vi "UHR-Fleezers Control (host) -Leonardo 04-2018 V1.vi"(0 "Tab Control":T5(tab)=enum."Trap Control (RF)") -> ()   [LabVIEW 2013] (continued)
                workers-P: _ -> [_]
                n1854 = Add Array Elements(numeric array=w3564) -> (sum=w3563:dbl)
              }
              n1855 = Select(t=w3550, s=w3551, f=w3549) -> (s? t:f=w3548:dbl)
              n1856 = Divide(x=w3555, y=w3548) -> (x/y=w3553:dbl[])
              n1857 = Bundle By Name(cluster=w3554, "magnitude"=w3553) -> (w3552:cluster{"f0":dbl, "df":dbl, "magnitude":dbl[]})
            }
          }
        }
        n1858 = case shown="True" w3494 {
          tunnel: w3495 -> [w3526 w3532]
          tunnel: [w3526 w3527] -> w3493
          frame False {
          }
          frame True {
            n1859 = Array Subset(array=w3532, index (row)=0 ("index"), length (row)=4 ("length"), index (col)=0 ("index"), length (col)=1 ("length")) -> (w3527:T47)
          }
        }
        n1860 = feedback-in #9(w3493) -> ()
        n1861 = Split 1D Array(array=w3507, index=2) -> (first subarray=→"FFT 1":cluster{"f0":dbl, "df":dbl, "magnitude":dbl[]}[], second subarray=→"FFT 2":cluster{"f0":dbl, "df":dbl, "magnitude":dbl[]}[])
      }
    }
    n1862 = Index Array(array=w2389, index=1) -> (element=w2397:waveform(dbl))
    n1863 = case "For displaying the high resolution display (no downsampling)" shown="True" w2453 {
      tunnel: w2416 -> [_ w2735]
      frame False {
      }
      frame True {
        n1864 = Index Array(array=w2735, index="High Res. Display") -> (element=w2736:waveform(dbl))
        n1865 = call <vilib>:"Std Deviation and Variance.vi"("X"=w2736) -> ("mean"=w2743:dbl, "standard deviation"=w2748:dbl)  [unwired: 1 in, 1 out]
        "Mean Intensity" <- w2743
        "Sigma" <- w2748
        n1866 = Subtract(x=w2736, y=w2743) -> (x-y=w2742:waveform(dbl))
        n1867 = Select(t=w2742, s="Subtract mean", f=w2736) -> (s? t:f=→"1 Channel":waveform(dbl))
        n1868 = Divide(x=w2748, y=w2743) -> (x/y=→"Sigma/Mean":dbl)
        n1869 = feedback #10(1) -> (w2737:i32)
        n1870 = Greater Or Equal?(x=w2737, y="Slow mean N ave.") -> (x >= y?=w2750:bool)
        n1871 = Increment(x=w2737) -> (x+1=w2752:i32)
        n1872 = Select(t=1, s=w2750, f=w2752) -> (s? t:f=w2739:i32)
        n1873 = feedback-in #10(w2739) -> ()
        n1874 = feedback #11() -> (w2740:waveform(dbl))  [unwired: 1 out]
        n1875 = case shown="Default" w2737 {
          tunnel: [w2755 w2758] -> w2741
          tunnel: w2740 -> [w2757 _]
          tunnel: w2736 -> [w2756 w2758]
          frame Default {
            n1876 = call-poly <vilib>:"Append Waveforms.vi"("waveform B"=w2756, "waveform A"=w2757) -> ("waveform out"=w2755:waveform(dbl))  [unwired: 1 in, 8 out]
          }
          frame 1 {
          }
        }
        n1877 = feedback-in #11(w2741) -> ()
        n1878 = case shown="True" w2750 {
          tunnel: w2741 -> [_ w2754]
          frame False {
          }
          frame True {
            n1879 = call-poly <vilib>:"Mean.vi"("X"=w2754) -> ("mean"=→"Slow mean":dbl)  [unwired: 1 out]
          }
        }
      }
    }
    n1880 = case "For plotting results of scanning MCL" shown="True" w2523 {
      tunnel: w2522 -> [_ w2875]
      tunnel: w2446 -> [_ w2971]
      tunnel: w2531 -> [_ _]
      tunnel: w2416 -> [_ w2945]
      tunnel: w2391 -> [_ w2876]
      tunnel: w2390 -> [_ w2849]
      frame False {
      }
      frame True {
        w2856 = u32 0 items=["Horizontal", "Vertical", "Central", "1st Diagonal", "2nd Diagonal"] ("Type of Symmetry")
        w2884 = u32 0 items=["Horizontal", "Vertical", "Central", "1st Diagonal", "2nd Diagonal"] ("Type of Symmetry")
        w2887 = u32 0 items=["Horizontal", "Vertical", "Central", "1st Diagonal", "2nd Diagonal"] ("Type of Symmetry")
        w2916 = u32 0 items=["Horizontal", "Vertical", "Central", "1st Diagonal", "2nd Diagonal"] ("Type of Symmetry")
        n1881 = Index Array(array=w2945, index=10) -> (element=w2951:waveform(dbl))
        n1882 = Index Array(array=w2945, index=11) -> (element=w2948:waveform(dbl))
        n1883 = local read "Cycles/step (MCL)"() -> (w2901:u64)
        n1884 = Index Array(array=w2945, index="Channel") -> (element=w2947:waveform(dbl))
        n1885 = Unbundle(w2849) -> ("New Image"=w2848:T3, "New Image"=w2847:T3, "New Image"=w2846:T3, "New Image"=w2845:T3)
        n1886 = Unbundle By Name(w2951) -> ("Y"=w2903:dbl[])
        n1887 = Unbundle By Name(w2948) -> ("Y"=w2905:dbl[])
        n1888 = Unbundle By Name(w2947) -> ("Y"=w2910:dbl[])
        n1889 = call "downsample 1D array - double.vi"("Ave N"=w2901, "Array In"=w2903) -> ("Array Out"=w2902:dbl[])  [unwired: 1 out]
        n1890 = call "downsample 1D array - double.vi"("Ave N"=w2901, "Array In"=w2905) -> ("Array Out"=w2904:dbl[])  [unwired: 1 out]
        n1891 = call "downsample 1D array - double.vi"("Ave N"=w2901, "Array In"=w2910) -> ("Array Out"=w2909:dbl[])  [unwired: 1 out]
        n1892 = feedback #12(w2971) -> (w2972:dbl[])
        n1893 = Build Array (concatenate)(w2972, w2971) -> (w2953:dbl[])
        n1894 = feedback #13(w2876) -> (w2878:dbl[])
        n1895 = Build Array (concatenate)(w2878, w2876) -> (w2877:dbl[])
        n1896 = local read "Scan steps (MCL)"() -> (w2858:u64)
        n1897 = Select(t=w2971, s=w2875, f=w2953) -> (s? t:f=w2957:dbl[])
        n1898 = feedback-in #12(w2957) -> ()
        n1899 = Select(t=w2876, s=w2875, f=w2877) -> (s? t:f=w2859:dbl[])
        n1900 = feedback-in #13(w2859) -> ()
        n1901 = local read "Scan lines (y)"() -> (w2844:u64)
        n1902 = local read "N APD Samp/step"() -> (w2860:dbl)
        n1903 = feedback #14(w2902) -> (w2959:dbl[])
        n1904 = Build Array (concatenate)(w2959, w2902) -> (w2950:dbl[])
        n1905 = feedback #15(w2909) -> (w2969:dbl[])
        n1906 = Build Array (concatenate)(w2969, w2909) -> (w2968:dbl[])
        n1907 = feedback #16(w2904) -> (w2961:dbl[])
        n1908 = Build Array (concatenate)(w2961, w2904) -> (w2962:dbl[])
        n1909 = Select(t=w2902, s=w2875, f=w2950) -> (s? t:f=w2906:dbl[])
        n1910 = feedback-in #14(w2906) -> ()
        n1911 = Select(t=w2909, s=w2875, f=w2968) -> (s? t:f=w2908:dbl[])
        n1912 = feedback-in #15(w2908) -> ()
        n1913 = Select(t=w2904, s=w2875, f=w2962) -> (s? t:f=w2907:dbl[])
        n1914 = feedback-in #16(w2907) -> ()
        n1915 = Multiply(x=w2858, y=u64 2) -> (x*y=w2843:u64)
        n1916 = call "integrate 1D array interval - double.vi"("Ave N"=w2860, "Array In"=w2859) -> ("Array Out"=w2871:dbl[])  [unwired: 1 out]
        n1917 = call "integrate 1D array interval - double.vi"("Ave N"=w2860, "Array In"=w2957) -> ("Array Out"=w2956:dbl[])  [unwired: 1 out]
        n1918 = Array Size(array=w2871) -> (size(s)=w2872:i32)
        n1919 = Array Size(array=w2956) -> (size(s)=w2958:i32)
        n1920 = Multiply(x=w2844, y=w2843) -> (x*y=w2874:u64)
        n1921 = Multiply(x=w2844, y=w2843) -> (x*y=w2966:u64)
        n1922 = call-poly <vilib>:"Mean.vi"("X"=w2906) -> ("mean"=w2890:dbl)  [unwired: 1 out]
        n1923 = Subtract(x=w2874, y=w2872) -> (x-y=w2865:u64)
        n1924 = call-poly <vilib>:"Mean.vi"("X"=w2908) -> ("mean"=w2895:dbl)  [unwired: 1 out]
        n1925 = call-poly <vilib>:"Mean.vi"("X"=w2907) -> ("mean"=w2893:dbl)  [unwired: 1 out]
        n1926 = call-poly <vilib>:"Mean.vi"("X"=w2871) -> ("mean"=w2862:dbl)  [unwired: 1 out]
        n1927 = Subtract(x=w2966, y=w2958) -> (x-y=w2900:u64)
        n1928 = call-poly <vilib>:"Mean.vi"("X"=w2956) -> ("mean"=w2897:dbl)  [unwired: 1 out]
        n1929 = Initialize Array(1.0 ("element"), w2865) -> (w2861:dbl[])
        n1930 = Initialize Array(1.0 ("element"), w2900) -> (w2891:dbl[])
        n1931 = Multiply(x=w2861, y=w2862) -> (x*y=w2863:dbl[])
        n1932 = Multiply(x=w2891, y=w2893) -> (x*y=w2894:dbl[])
        n1933 = Multiply(x=w2891, y=w2895) -> (x*y=w2896:dbl[])
        n1934 = Multiply(x=w2891, y=w2890) -> (x*y=w2892:dbl[])
        n1935 = Multiply(x=w2891, y=w2897) -> (x*y=w2898:dbl[])
        n1936 = Build Array (concatenate)(w2906, w2892) -> (w2960:dbl[])
        n1937 = Build Array (concatenate)(w2908, w2896) -> (w2964:dbl[])
        n1938 = Build Array (concatenate)(w2907, w2894) -> (w2963:dbl[])
        n1939 = Build Array (concatenate)(w2871, w2863) -> (w2873:dbl[])
        n1940 = Build Array (concatenate)(w2956, w2898) -> (w2965:dbl[])
        n1941 = Reshape Array(w2960, w2844, w2843) -> (w2926:dbl[][])
        n1942 = Reshape Array(w2873, w2844, w2843) -> (w2869:dbl[][])
        n1943 = Reshape Array(w2964, w2844, w2843) -> (w2918:dbl[][])
        n1944 = Reshape Array(w2963, w2844, w2843) -> (w2933:dbl[][])
        n1945 = Reshape Array(w2965, w2844, w2843) -> (w2943:dbl[][])
        n1946 = Array Subset(array=w2933, index (col)=0 ("index"), length (col)=w2858) -> (w2938:dbl[][])  [unwired: 2 in]
        n1947 = Array Subset(array=w2933, index (col)=w2858) -> (w2936:dbl[][])  [unwired: 3 in]
        n1948 = Array Subset(array=w2918, index (col)=0 ("index"), length (col)=w2858) -> (w2924:dbl[][])  [unwired: 2 in]
        n1949 = Array Subset(array=w2918, index (col)=w2858) -> (w2922:dbl[][])  [unwired: 3 in]
        n1950 = Array Subset(array=w2869, index (col)=0 ("index"), length (col)=w2858) -> (w2868:dbl[][])  [unwired: 2 in]
        n1951 = Array Subset(array=w2869, index (col)=w2858) -> (w2866:dbl[][])  [unwired: 3 in]
        n1952 = Array Subset(array=w2943, index (col)=0 ("index"), length (col)=w2858) -> (w2942:dbl[][])  [unwired: 2 in]
        n1953 = Array Subset(array=w2943, index (col)=w2858) -> (w2940:dbl[][])  [unwired: 3 in]
        n1954 = Array Subset(array=w2926, index (col)=0 ("index"), length (col)=w2858) -> (w2931:dbl[][])  [unwired: 2 in]
        n1955 = Array Subset(array=w2926, index (col)=w2858) -> (w2929:dbl[][])  [unwired: 3 in]
        n1956 = for {
          tunnel: w2938 -> [w2980] mode=indexing
          tunnel: [w2979] -> w2937 mode=indexing
          workers-P: _ -> [_]
          n1957 = Reverse 1D Array(array=w2980) -> (reversed array=w2979:dbl[])
        }
        n1958 = for {
          tunnel: w2924 -> [w2976] mode=indexing
          tunnel: [w2975] -> w2923 mode=indexing
          workers-P: _ -> [_]
          n1959 = Reverse 1D Array(array=w2976) -> (reversed array=w2975:dbl[])
        }
        n1960 = for {
          tunnel: w2868 -> [w2974] mode=indexing
          tunnel: [w2973] -> w2867 mode=indexing
          workers-P: _ -> [_]
          n1961 = Reverse 1D Array(array=w2974) -> (reversed array=w2973:dbl[])
        }
        n1962 = for {
          tunnel: w2942 -> [w2982] mode=indexing
          tunnel: [w2981] -> w2941 mode=indexing
          workers-P: _ -> [_]
          n1963 = Reverse 1D Array(array=w2982) -> (reversed array=w2981:dbl[])
        }
        n1964 = for {
          tunnel: w2931 -> [w2978] mode=indexing
          tunnel: [w2977] -> w2930 mode=indexing
          workers-P: _ -> [_]
          n1965 = Reverse 1D Array(array=w2978) -> (reversed array=w2977:dbl[])
        }
        n1966 = Index Array(array=w2943, index (row)=0) -> (element=→"Waveform Graph":dbl[])  [unwired: 1 in]
        n1967 = Add(x=w2937, y=w2936) -> (x+y=w2935:dbl[][])
        n1968 = Add(x=w2923, y=w2922) -> (x+y=w2921:dbl[][])
        n1969 = Add(x=w2867, y=w2866) -> (x+y=w2851:dbl[][])
        n1970 = Add(x=w2941, y=w2940) -> (x+y=w2915:dbl[][])
        n1971 = Add(x=w2930, y=w2929) -> (x+y=w2928:dbl[][])
        n1972 = Divide(x=w2921, y=2) -> (x/y=w2919:dbl[][])
        n1973 = Divide(x=w2935, y=2) -> (x/y=w2880:dbl[][])
        n1974 = Divide(x=w2928, y=2) -> (x/y=w2882:dbl[][])
        n1975 = To Single Precision Float(number=w2915) -> (single precision float=w2914:sgl[][])
        n1976 = Transpose 2D Array(2D array=w2919) -> (transposed array=→"Data map":dbl[][])
        n1977 = To Single Precision Float(number=w2851) -> (single precision float=w2855:sgl[][])
        n1978 = To Single Precision Float(number=w2880) -> (single precision float=w2886:sgl[][])
        n1979 = To Single Precision Float(number=w2882) -> (single precision float=w2883:sgl[][])
        n1980 = call "IMAQ ArrayToImage"("Image Pixels (Float)"=w2914, "Image"=w2848) -> ("Image Out"=w2917:T3)  [unwired: 8 in, 1 out]
        n1981 = call "IMAQ ArrayToImage"("Image Pixels (Float)"=w2855, "Image"=w2847) -> ("Image Out"=w2857:T3)  [unwired: 8 in, 1 out]
        n1982 = call "IMAQ ArrayToImage"("Image Pixels (Float)"=w2886, "Image"=w2846) -> ("Image Out"=w2888:T3)  [unwired: 8 in, 1 out]
        n1983 = call "IMAQ ArrayToImage"("Image Pixels (Float)"=w2883, "Image"=w2845) -> ("Image Out"=w2885:T3)  [unwired: 8 in, 1 out]
        n1984 = call "IMAQ Symmetry"("Type of Symmetry"=w2916, "Image Src"=w2917) -> ("Image Dst Out"=w2912:T3)  [unwired: 3 in, 1 out]
        n1985 = call "IMAQ Symmetry"("Type of Symmetry"=w2856, "Image Src"=w2857) -> ("Image Dst Out"=w2853:T3)  [unwired: 3 in, 1 out]
        n1986 = call "IMAQ Symmetry"("Type of Symmetry"=w2887, "Image Src"=w2888) -> ("Image Dst Out"=→"Detection Laser X":T3)  [unwired: 3 in, 1 out]
        n1987 = call "IMAQ Symmetry"("Type of Symmetry"=w2884, "Image Src"=w2885) -> ("Image Dst Out"=→"Detection Laser Y":T3)  [unwired: 3 in, 1 out]
        n1988 = call "IMAQ Set Simple Calibration"("Calibration Axis Info"=T37 {"Origin Pixel"={"X"=0.0, "Y"=0.0}, "Angle Relative to Horizontal (deg)"=0.0, "Axis Reference"=0}, "Grid Descriptor"=T38 {"X Step"=0.3, "Y Step"=0.3, "Unit"=enum."Undefined"}, "Image"=w2912) -> ("Calibrated Image"=→"APD 1":T3)  [unwired: 7 in, 1 out]
        n1989 = call "IMAQ Set Simple Calibration"("Calibration Axis Info"=T37 {"Origin Pixel"={"X"=0.0, "Y"=0.0}, "Angle Relative to Horizontal (deg)"=0.0, "Axis Reference"=0}, "Grid Descriptor"=T38 {"X Step"=0.3, "Y Step"=0.3, "Unit"=enum."Undefined"}, "Image"=w2853) -> ("Calibrated Image"=→"APD 2":T3)  [unwired: 7 in, 1 out]
      }
    }
    n1990 = Subtract(x=w2397, y="APD 2 Offset") -> (x-y=w2394:waveform(dbl))
    n1991 = Subtract(x=w2399, y="APD 1 Offset") -> (x-y=w2395:waveform(dbl))
    n1992 = Index Array(array=w2414, index=3) -> (element=w2473:waveform(dbl))
    n1993 = Index Array(array=w2414, index=6) -> (element=w2470:waveform(dbl))
    n1994 = Build Array(w2395, w2394) -> (→"APD Chart":waveform(dbl)[])
    n1995 = Array Size(array=w2463) -> (size(s)=w2511:i32)
    n1996 = call <vilib>:"Std Deviation and Variance.vi"("X"=w2407) -> ("standard deviation"=w2406:dbl)  [unwired: 1 in, 2 out]
    n1997 = Add Array Elements(numeric array=w2407) -> (sum=w2409:u32)
    n1998 = Add Array Elements(numeric array=w2463) -> (sum=w2521:u32)
    n1999 = call <vilib>:"Std Deviation and Variance.vi"("X"=w2463) -> ("standard deviation"=w2462:dbl)  [unwired: 1 in, 2 out]
    n2000 = Divide(x=w2406, y=w2405) -> (x/y=w2402:dbl)
    "Rate sigma (Hz) 2" <- w2402
    n2001 = Multiply(x=w2405, y=w2511) -> (x*y=w2408:dbl)
    "Int. Time (s)" <- w2408
    n2002 = Divide(x=w2409, y=w2408) -> (x/y=w2403:dbl)
    "APD 2 Rate (Hz)" <- w2403
    n2003 = Divide(x=w2521, y=w2408) -> (x/y=w2460:dbl)
    "APD 1 Rate (Hz)" <- w2460
    n2004 = Divide(x=w2462, y=w2405) -> (x/y=w2461:dbl)
    "Rate sigma (Hz)" <- w2461
    n2005 = Divide(x=w2402, y=w2403) -> (x/y=→"Sigma/Mean 2":dbl)
    n2006 = Divide(x=w2461, y=w2460) -> (x/y=→"Sigma/Mean":dbl)
    n2007 = case shown="2" "Calibration" {
      tunnel: "T1 alpha_x (nm/V)" -> [_ w2811 w2832]
      tunnel: "T1 kappa_x (pN/nm)" -> [_ _ w2822]
      tunnel: "T2 alpha_x (nm/V)" -> [_ w2810 w2830]
      tunnel: "T2 kappa_x (pN/nm)" -> [_ _ w2823]
      tunnel: w2473 -> [w2793 w2808 w2828]
      tunnel: w2470 -> [w2792 w2806 w2826]
      tunnel: [w2793 w2805 w2825] -> w2263
      tunnel: [w2792 w2804 w2824] -> w2269
      tunnel: ["T1 X (V)" ("Label.Text") "T1 X (nm)" ("Label.Text") "T1 X (pN)" ("Label.Text")] -> w2491
      tunnel: ["T2 X (V)" ("Label.Text") "T2 X (nm)" ("Label.Text") "T2 X (pN)" ("Label.Text")] -> w2490
      tunnel: ["Position (V)" ("Label.Text") "Position (nm)" ("Label.Text") "Force (pN)" ("Label.Text")] -> w2492
      tunnel: w2472 -> [_ w2796 w2815]
      tunnel: w2474 -> [_ w2799 w2817]
      tunnel: ["Mean (V)" ("Label.Text") "Mean (nm)" ("Label.Text") "Mean (pN)" ("Label.Text")] -> w2487
      tunnel: ["Difference (V)" ("Label.Text") "Difference (nm)" ("Label.Text") "Difference (pN)" ("Label.Text")] -> w2422
      frame 0, Default {
      }
      frame 1 {
        # "position"
        n2008 = Unbundle By Name(w2808) -> ("Y"=w2812:dbl[])
        n2009 = Unbundle By Name(w2806) -> ("Y"=w2797:dbl[])
        n2010 = Subtract(x=w2812, y=w2799) -> (x-y=w2800:dbl[])
        n2011 = Subtract(x=w2797, y=w2796) -> (x-y=w2798:dbl[])
        n2012 = Multiply(x=w2798, y=w2810) -> (x*y=w2807:dbl[])
        n2013 = Multiply(x=w2811, y=w2800) -> (x*y=w2809:dbl[])
        n2014 = Bundle By Name(cluster=w2806, "Y"=w2807) -> (w2804:waveform(dbl))
        n2015 = Bundle By Name(cluster=w2808, "Y"=w2809) -> (w2805:waveform(dbl))
      }
      frame 2 {
        # "force"
        n2016 = Unbundle By Name(w2828) -> ("Y"=w2833:dbl[])
        n2017 = Unbundle By Name(w2826) -> ("Y"=w2831:dbl[])
        n2018 = Subtract(x=w2831, y=w2815) -> (x-y=w2816:dbl[])
        n2019 = Subtract(x=w2833, y=w2817) -> (x-y=w2818:dbl[])
        n2020 = Compound Arithmetic op=MULTIPLY(w2816, w2830, w2823) -> (w2827:dbl[])
        n2021 = Compound Arithmetic op=MULTIPLY(w2822, w2832, w2818) -> (w2829:dbl[])
        n2022 = Bundle By Name(cluster=w2826, "Y"=w2827) -> (w2824:waveform(dbl))
        n2023 = Bundle By Name(cluster=w2828, "Y"=w2829) -> (w2825:waveform(dbl))
      }
    }
    n2024 = feedback-in #17("Calibration") -> ()
    n2025 = feedback #17(u16 1 ("Calibration")) -> (w2494:u16)
    n2026 = local read "Trap 2 Bead Size (nm)"() -> (w2302:dbl)
    n2027 = local read "Trap 1 Bead Size (nm)"() -> (w2301:dbl)
    n2028 = local read "AOM X Cal (nm/MHz)"() -> (w2299:dbl)
    n2029 = local read "Trap Delta (MHz)"() -> (w2298:dbl)
    n2030 = Not Equal?(x=w2494, y="Calibration") -> (x != y?=w2451:bool)
    n2031 = Multiply(x=w2299, y=w2298) -> (x*y=w2303:dbl)
    n2032 = Unbundle By Name(w2263) -> ("Y"=w2268:dbl[])
    n2033 = Unbundle By Name(w2269) -> ("Y"=w2267:dbl[])
    n2034 = Add(x=w2302, y=w2301) -> (x+y=w2305:dbl)
    n2035 = case shown="False" "Negate trap 2 force" {
      tunnel: [-1.0 1.0] -> w2480
      frame False {
      }
      frame True {
      }
    }
    n2036 = Unbundle By Name(w2473) -> ("Y"=w2476:dbl[])
    n2037 = Unbundle By Name(w2470) -> ("Y"=w2479:dbl[])
    n2038 = Divide(x=w2305, y=2.0) -> (x/y=w2300:dbl)
    n2039 = Subtract(x=w2268, y=w2267) -> (x-y=w2265:dbl[])
    n2040 = Subtract(x=w2476, y=w2474) -> (x-y=w2477:dbl[])
    n2041 = Subtract(x=w2479, y=w2472) -> (x-y=w2478:dbl[])
    n2042 = Divide(x=w2265, y=2.0) -> (x/y=w2264:dbl[])
    n2043 = Multiply(x=w2478, y="T2 alpha_x (nm/V)") -> (x*y=w2469:dbl[])
    n2044 = Multiply(x="T1 alpha_x (nm/V)", y=w2477) -> (x*y=w2468:dbl[])
    n2045 = Multiply(x=w2269, y=w2480) -> (x*y=w2481:waveform(dbl))
    n2046 = Bundle By Name(cluster=w2263, "Y"=w2264) -> (w2262:waveform(dbl))
    n2047 = case shown="True" "Read Lateness and Rel Phase" {
      tunnel: w2275 -> [w2759 w2781]
      tunnel: w2314 -> [w2760 w2780]
      tunnel: [w2759 w2779] -> w2466
      tunnel: [w2760 w2778] -> w2465
      frame False {
      }
      frame True {
        n2048 = xnode "Read/Write Control"("FPGA VI Reference In"=w2781, "error in"=w2780) -> ("FPGA VI Reference Out"=w2779:T20, "error out"=w2778:errorcluster, "GI Relative phase"=→"GI relative phase":i16, "Relative phase"=→"Relative phase (AI1)":i16, "AI Late Counter"=→"Late Counter (AI1)":u8, "GI Late Counter"=→"GI Late Counter":u8, "MCL Late Counter"=→"MCL Late Counter":u8, "MCL Relative Phase"=→"Relative Phase (MCL)":i16, "APD Acq Relative Phase"=→"APD Acq Relative Phase":i16, "APD 1 Gate Relative Phase"=→"APD 1 Gate Relative Phase":i16, "APD 2 Gate Relative Phase"=→"APD 2 Gate Relative Phase":i16, "APD Acq Late Counter"=→"APD Acq Late Counter":u16, "APD 1 Gate Late Counter"=→"APD 1 Gate Late Counter":u8, "APD 2 Gate Late Counter"=→"APD 2 Gate Late Counter":u8, "Green FB Relative Phase"=→"Relative phase (Green FB)":i16, "GI Relative phase"=→"GI relative phase 2":i16, "GI Late Counter 2"=→"GI Late Counter 2":u16, "Trap Pos FIFO Timeout"=→"Trap Pos FIFO Timeout":u16, "Trap AI FIFO Timeout"=→"Trap AI FIFO Timeout":u16)
      }
    }
    n2049 = Subtract(x=w2469, y=w2468) -> (x-y=w2297:dbl[])
    n2050 = call-poly <vilib>:"Mean.vi"("X"=w2297) -> ("mean"=w2304:dbl)  [unwired: 1 out]
    n2051 = Add(x=w2303, y=w2304) -> (x+y=w2307:dbl)
    n2052 = Subtract(x=w2307, y=w2300) -> (x-y=→"Tether Extension (nm, calculated)":dbl)
    n2053 = Unbundle By Name(w2269) -> ("Y"=w2260:dbl[])
    n2054 = Unbundle By Name(w2263) -> ("Y"=w2261:dbl[])
    n2055 = Build Array(w2263, w2481, w2262) -> (→"Force":waveform(dbl)[])
    n2056 = Subtract(x=w2297, y="Offset (nm)") -> (x-y=w2441:dbl[])
    n2057 = call-poly <vilib>:"Mean.vi"("X"=w2260) -> ("mean"=w2258:dbl)  [unwired: 1 out]
    "T2 X" <- w2258
    n2058 = call-poly <vilib>:"Mean.vi"("X"=w2261) -> ("mean"=w2259:dbl)  [unwired: 1 out]
    "T1 X" <- w2259
    n2059 = Subtract(x=w2261, y=w2260) -> (x-y=w2443:dbl[])
    n2060 = Bundle By Name(cluster=w2473, "Y"=w2441) -> (w2413:waveform(dbl))
    "Bead Separation" <- w2413
    n2061 = Divide(x=w2443, y=2.0) -> (x/y=→"Vec Mean of T1 T2":dbl[])
    n2062 = case shown="True" w2451 {
      tunnel: w2492 -> [_ w2786]
      tunnel: w2491 -> [_ w2785]
      tunnel: w2490 -> [_ w2784]
      tunnel: w2487 -> [_ w2783]
      tunnel: w2422 -> [_ w2782]
      frame False {
      }
      frame True {
        n2063 = property on="Force" class="WFChart (strict)"("YScale.NameLbl.Text"=w2786) -> ()  [unwired: 2 in, 2 out]
        n2064 = property on="T2 X" class="DigNum (strict)"("Caption.Text"=w2784) -> ()  [unwired: 2 in, 2 out]
        n2065 = property on="T1 X" class="DigNum (strict)"("Caption.Text"=w2785) -> ()  [unwired: 2 in, 2 out]
        n2066 = property on="Mean" class="DigNum (strict)"("Caption.Text"=w2783) -> ()  [unwired: 2 in, 2 out]
        n2067 = property on="Difference" class="DigNum (strict)"("Caption.Text"=w2782) -> ()  [unwired: 2 in, 2 out]
      }
    }
    n2068 = local read "Tether"() -> (w2445:bool)
    n2069 = Subtract(x=w2259, y=w2258) -> (x-y=w2489:dbl)
    n2070 = Add(x=w2259, y=w2258) -> (x+y=→"Difference":dbl)
    n2071 = feedback #18(w2441) -> (w2440:dbl[])
    n2072 = Divide(x=w2489, y=2.0) -> (x/y=w2272:dbl)
    "Mean" <- w2272
    n2073 = case shown="True" w2445 {
      tunnel: w2272 -> [_ w2718]
      frame False {
      }
      frame True {
        n2074 = Greater?(x="Lost Tether Alarm Threshold (pN)", y=w2718) -> (0:w2716:bool)
        n2075 = case shown="True" w2716 {
          frame False {
          }
          frame True {
            n2076 = flat-sequence {
              frame #0 {
                # "stop only if saving"
                n2077 = local read "Saving..."() -> (w2731:bool)
                n2078 = And(x=w2731, y="TA Cancel Save?") -> (x .and. y?=w2730:bool)
                n2079 = local write "Stop Saving"(w2730) -> ()
              }
              frame #1 {
                n2080 = case shown="True" "TA Green Off?" {
                  frame False {
                  }
                  frame True {
                    w2734 = FALSE ("Fl. Triggered...")
                    n2081 = local write "Fl. Triggered..."(w2734) -> ()
                    n2082 = property on="Green Laser ON/Interlacing" class="Bool (strict)"("Val(Sgnl)"=w2734) -> ()  [unwired: 2 in, 2 out]
                  }
                }
              }
            }
            n2083 = local read "Time tether formed"() -> (w2725:timestamp)
            n2084 = Get Date/Time In Seconds() -> (seconds since 1Jan1904=w2726:timestamp)
            n2085 = Subtract(x=w2726, y=w2725) -> (x-y=w2724:dbl)
            n2086 = Number To Decimal String(number=w2724) -> (decimal integer string=w2721:string)  [unwired: 1 out]
            n2087 = local read "Messages"() -> (w2728:string)
            n2088 = call <vilib>:"Beep.vi"() -> ()  [unwired: 3 in, 9 out]
            n2089 = Concatenate Strings("Lost tether (" ("Message to add"), w2721, " s)." ("string")) -> (w2723:string)
            n2090 = local write "Tether"(FALSE ("Tether")) -> ()
            n2091 = call "Update messages.vi"("Message to add"=w2723, "Old message string"=w2728) -> ("New message string"=w2727:string)
            n2092 = local write "Messages"(w2727) -> ()
            n2093 = property on="Trap Pos. FB ON" class="Bool (strict)"("Val(Sgnl)"=FALSE ("Value (Signaling)")) -> ()  [unwired: 2 in, 2 out]
          }
        }
      }
    }
    n2094 = Build Array (concatenate)(w2441, w2440) -> (w2439:dbl[])
    n2095 = Split 1D Array(array=w2439, index=w2325) -> (first subarray=w2435:dbl[])  [unwired: 1 out]
    n2096 = feedback-in #18(w2435) -> ()
    n2097 = call-poly <vilib>:"Mean.vi"("X"=w2435) -> ("mean"=w2434:dbl)  [unwired: 1 out]
    "Bead Mean (nm)" <- w2434
    n2098 = Subtract(x=w2435, y=w2434) -> (x-y=w2433:dbl[])
    n2099 = Square(x=w2433) -> (x^2=w2432:dbl[])
    n2100 = case shown="True" "Semi Passive ON" {
      tunnel: "Semi Passive mode" -> [_ w2599]
      tunnel: "Jump Force (pN)" -> [_ w2598]
      tunnel: w2272 -> [_ w2597]
      frame False {
      }
      frame True {
        n2101 = case shown="\"Use Feedback\"" w2599 {
          tunnel: w2598 -> [_ w2602 w2618]
          tunnel: w2597 -> [_ w2601 w2617]
          frame "None" {
          }
          frame "Use Feedback" {
            n2102 = local read "Target Force (pN)"() -> (w2604:dbl)
            n2103 = Less?(x=w2602, y=w2604) -> (x < y?=w2603:bool)
            n2104 = case shown="True" w2603 {
              tunnel: w2602 -> [w2611 w2614]
              tunnel: w2601 -> [w2610 w2613]
              tunnel: [w2609 w2612] -> w2600
              frame False {
                n2105 = Less?(x=w2611, y=w2610) -> (x < y?=w2609:bool)
              }
              frame True {
                n2106 = Greater?(x=w2614, y=w2613) -> (0:w2612:bool)
              }
            }
            n2107 = case shown="True" w2600 {
              frame False {
                n2108 = local read "Trap Pos. FB ON"() -> (w2605:bool)
                n2109 = case shown="True" w2605 {
                  frame False {
                  }
                  frame True {
                    n2110 = property on="Trap Pos. FB ON" class="Bool (strict)"("Val(Sgnl)"=FALSE) -> ()  [unwired: 2 in, 2 out]
                  }
                }
              }
              frame True {
                n2111 = local read "Trap Pos. FB ON"() -> (w2607:bool)
                n2112 = case shown="False" w2607 {
                  frame False {
                    n2113 = property on="Trap Pos. FB ON" class="Bool (strict)"("Val(Sgnl)"=TRUE) -> ()  [unwired: 2 in, 2 out]
                  }
                  frame True {
                  }
                }
              }
            }
          }
          frame "Sharp Jump" {
            n2114 = local read "Target Force (pN)"() -> (w2620:dbl)
            n2115 = Greater?(x=w2618, y=w2620) -> (0:w2619:bool)
            n2116 = case shown="True" w2619 {
              tunnel: w2618 -> [w2635 w2639]
              tunnel: w2617 -> [w2636 w2638]
              tunnel: [w2634 w2637] -> w2616
              frame False {
                n2117 = Greater?(x=w2636, y=w2635) -> (0:w2634:bool)
              }
              frame True {
                n2118 = Less?(x=w2639, y=w2638) -> (x < y?=w2637:bool)
              }
            }
            n2119 = Subtract(x=w2618, y=w2620) -> (x-y=w2615:dbl)
            n2120 = case shown="True" w2616 {
              tunnel: w2615 -> [_ w2626]
              frame False {
              }
              frame True {
                n2121 = local read "T1 kappa_x (pN/nm)"() -> (w2631:dbl)
                n2122 = local read "T2 kappa_x (pN/nm)"() -> (w2632:dbl)
                n2123 = Reciprocal(x="DNA stiffness (pN / nm)") -> (1/x=w2628:dbl)
                n2124 = Reciprocal(x=w2631) -> (1/x=w2630:dbl)
                n2125 = Reciprocal(x=w2632) -> (1/x=w2629:dbl)
                n2126 = Compound Arithmetic op=ADD(w2630, w2629, w2628) -> (w2627:dbl)
                n2127 = local read "AOM X Cal (nm/MHz)"() -> (w2625:dbl)
                n2128 = Multiply(x=w2627, y=w2626) -> (x*y=w2624:dbl)
                n2129 = local read "Trap Delta (MHz)"() -> (w2622:dbl)
                n2130 = Divide(x=w2624, y=w2625) -> (x/y=w2623:dbl)
                n2131 = Subtract(x=w2622, y=w2623) -> (x-y=w2621:dbl)
                n2132 = property on="Trap Delta (MHz)" class="DigNum (strict)"("Val(Sgnl)"=w2621) -> ()  [unwired: 2 in, 2 out]
              }
            }
          }
        }
      }
    }
    n2133 = call-poly <vilib>:"Mean.vi"("X"=w2432) -> ("mean"=w2431:dbl)  [unwired: 1 out]
    n2134 = Square Root(x=w2431) -> (sqrt(x)=w2430:dbl)
    n2135 = Multiply(x=10.0, y=w2430) -> (x*y=→"RMS (Ang)":dbl)
    n2136 = xnode "Read/Write Control"("FPGA VI Reference In"=w2466, "error in"=w2465) -> ("FPGA VI Reference Out"=w2575:T20, "error out"=w2569:errorcluster, "AI2 Y Sum Set 1"=w2565:i16, "AI2 Y Sum Set 2"=w2564:i16, "AI1 X Set 1"=w2359:fxp<+/-,16,1>, "AI1 X Set 2"=w2358:fxp<+/-,16,1>, "Trap Pos FB Int Signal"=→"Trap Pos FB Int Signal":fxp<+/-,24,9>, "Trap Pos FB Int-Norm Signal"=→"Trap Pos FB Int-Norm Signal":fxp<+/-,16,1>, "Trap Pos FB Action"=w2352:i64, "Scanning"=→"AOD Scanning":bool, "Scan I"=→"AOD Scan I":u64, "Scanning MCL"=w2567:bool, "Scan I (MCL)"=→"MCL Scan I":u64, "Green FB Signals"=w2506:T48, "BD1 amplitude 1 out"=w2257:u16, "BD1 amplitude 2 out"=w2242:u16)  [unwired: 1 out]
    "MCL Scanning" <- w2567
    "Trap Pos FB Action" <- w2352
    n2137 = local read "AI2 (V)"() -> (w2566:cluster{"Set 1":dbl, "Set 2":dbl})
    n2138 = Bundle By Name(cluster=w2566, "Set 1"=w2565, "Set 2"=w2564) -> (w2562:cluster{"Set 1":dbl, "Set 2":dbl})
    n2139 = Divide(x=w2352, y=327.67) -> (x/y=→"Action (%)":dbl)
    n2140 = local read "Trap X (AI1)"() -> (w2372:T1)
    n2141 = Divide(x=w2562, y=3276.7) -> (x/y=w2561:cluster{"Set 1":dbl, "Set 2":dbl})
    n2142 = local write "AI2 (V)"(w2561) -> ()
    n2143 = Bundle(cluster=w2372, "Trap 1"=w2359, "Trap 2"=w2358) -> (→"Trap X (AI1)":T1)
    n2144 = Scale By Power Of 2(n=i16 12, x=ext 1.0) -> (x*2^n=w2253:ext)
    n2145 = Subtract(x=w2253, y=ext 1.0) -> (x-y=w2250:ext)
    n2146 = Divide(x=w2506, y=3276.7) -> (x/y=w2502:T49)
    n2147 = Multiply(x=w2257, y=ext 100.0) -> (x*y=w2251:ext)
    n2148 = Unbundle By Name(w2502) -> ("Green FB Ch 0"=w2505:dbl, "Green FB Ch 1"=w2504:dbl, "Green FB Ch 2"=w2503:dbl)
    n2149 = local read "All FB On/Off"() -> (w2241:bool)
    n2150 = Divide(x=w2251, y=w2250) -> (x/y=w2240:ext)
    "Trap 1 amplitude" <- w2240
    n2151 = Scale By Power Of 2(n=i16 12, x=ext 1.0) -> (x*2^n=w2246:ext)
    n2152 = Subtract(x=w2246, y=ext 1.0) -> (x-y=w2249:ext)
    n2153 = Multiply(x=w2242, y=ext 100.0) -> (x*y=w2248:ext)
    n2154 = Divide(x=w2505, y=w2503) -> (x/y=w2501:dbl)
    n2155 = Divide(x=w2504, y=w2503) -> (x/y=w2500:dbl)
    n2156 = flat-sequence "To save data" {
      tunnel: [w3615] -> w2586
      tunnel: [w3616] -> w2585
      tunnel: w2537 -> [w3609]
      tunnel: w2437 -> [w3613]
      tunnel: ["Save Calibration"] -> w2558
      tunnel: w2555 -> [w3612]
      tunnel: [w3605] -> w2554
      tunnel: [w3602] -> w2553
      tunnel: [w3599] -> w2552
      tunnel: w2536 -> [w3601]
      tunnel: w2449 -> [w3595]
      tunnel: [w3595] -> w2448
      tunnel: ["Start Saving"] -> w2415
      tunnel: [w3589] -> w2341
      tunnel: [w3588] -> w2340
      tunnel: w2586 -> [w3850]
      tunnel: w2585 -> [w3849]
      tunnel: w2342 -> [w3848]
      tunnel: w2558 -> [w3847]
      tunnel: w2554 -> [w3845]
      tunnel: w2553 -> [w3844]
      tunnel: w2552 -> [w3843]
      tunnel: w2424 -> [w3842]
      tunnel: w2458 -> [w3841]
      tunnel: w2448 -> [w3840]
      tunnel: w2415 -> [w3839]
      tunnel: w2413 -> [w3838]
      tunnel: w2389 -> [w3837]
      tunnel: w2341 -> [w3836]
      tunnel: w2340 -> [w3835]
      tunnel: w2339 -> [w3834]
      frame #0 {
        n2157 = Or(x="Save N Sets", y="Start Saving") -> (x .or. y?=w3596:bool)
        n2158 = To Double Precision Float(number=w3612) -> (double precision float=w3606:dbl)
        n2159 = Build Array(w3596, "Save Calibration", w3609, w3601) -> (w3611:bool[])
        n2160 = Compound Arithmetic op=OR("Save Calibration", w3609, w3596, w3601) -> (w3614:bool)
        n2161 = Boolean Array To Number(Boolean array=w3611) -> (number=w3608:u32)
        n2162 = feedback #19(FALSE ("Save APD Data\nwith Trap Data")) -> (w3590:bool)
        n2163 = feedback #20(refnum<k0> refnum) -> (w3617:refnum<file>)
        n2164 = feedback #21(refnum<k0> refnum) -> (w3592:refnum<file>)
        n2165 = feedback #22(FALSE ("Save APD Data\nwith Trap Data")) -> (w3600:bool)
        n2166 = feedback #23(refnum<k0> refnum) -> (w3603:refnum<file>)
        n2167 = feedback #24(0) -> (w3619:i32)
        n2168 = feedback #25() -> (w3607:u32)  [unwired: 1 out]
        n2169 = case shown="True" w3614 {
          tunnel: [w3626 1] -> w3615
          tunnel: w3619 -> [w3628 _]
          tunnel: [w3627 w3646] -> w3616
          tunnel: w3617 -> [w3627 _]
          tunnel: w3613 -> [_ w3666]
          tunnel: w3606 -> [_ w3664]
          tunnel: w3608 -> [_ w3667]
          tunnel: [w3625 w3645] -> w3605
          tunnel: w3607 -> [w3625 _]
          tunnel: [w3624 w3643] -> w3602
          tunnel: w3603 -> [w3624 _]
          tunnel: [w3623 w3642] -> w3599
          tunnel: w3600 -> [w3623 _]
          tunnel: "Start Saving" -> [_ w3640]
          tunnel: w3595 -> [_ w3639]
          tunnel: [w3622 w3630] -> w3588
          tunnel: w3592 -> [w3622 _]
          tunnel: [w3621 w3629] -> w3589
          tunnel: w3590 -> [w3621 _]
          frame False {
            n2170 = Increment(x=w3628) -> (x+1=w3626:i32)
          }
          frame True {
            w3636 = FALSE ("Start Saving")
            w3641 = 9.0  # File Version
            w3649 = FALSE ("prepend array or string size? (T)")
            w3647 = T30."big-endian, network order" ("byte order (0:big-endian, network order)")
            # "write file headers"
            n2171 = local read "BD 1 Frequency 1 (MHz)"() -> (w3663:dbl)
            n2172 = local read "BD 2 Frequency 1 (MHz)"() -> (w3662:dbl)
            n2173 = local read "BD 1 Frequency 2 (MHz)"() -> (w3661:dbl)
            n2174 = local read "BD 2 Frequency 2 (MHz)"() -> (w3660:dbl)
            n2175 = local read "BD 1 Frequency 3 (MHz)"() -> (w3659:dbl)
            n2176 = local read "BD 2 Frequency 3 (MHz)"() -> (w3658:dbl)
            n2177 = Array Size(array=w3639) -> (size(s)=w3638:i32)
            n2178 = To Double Precision Float(number=w3638) -> (double precision float=w3637:dbl)
            n2179 = local write "Save Calibration"(w3636) -> ()
            n2180 = local write "Start Saving"(w3636) -> ()
            n2181 = Build Array("Save APD Data\nwith Trap Data", "Save Trap Pos. Data") -> (w3633:bool[])
            n2182 = Boolean Array To Number(Boolean array=w3633) -> (number=w3632:u32)
            n2183 = Build Array(w3663, w3662, w3661, w3660, w3659, w3658) -> (w3657:dbl[])
            n2184 = case shown="4" w3667 {
              tunnel: w3666 -> [w3738 w3758 w3774 w3812]
              tunnel: w3637 -> [w3743 w3765 w3794 w3831]
              tunnel: w3664 -> [w3742 w3764 w3793 w3830]
              tunnel: [w3739 w3760 w3785 w3822] -> w3655
              tunnel: [w3730 "Cal sets to save" w3775 w3813] -> w3645
              tunnel: w3657 -> [w3740 w3761 w3787 w3824]
              tunnel: "Save APD Data\nwith Trap Data" -> [w3737 _ w3771 w3810]
              tunnel: [w3737 w3752 w3771 w3810] -> w3642
              tunnel: w3641 -> [w3733 w3753 w3769 w3808]
              tunnel: w3640 -> [w3732 _ _ _]
              tunnel: [w3723 w3752 w3768 w3798] -> w3629
              tunnel: "Save Trap Pos. Data" -> [w3723 _ w3768 w3798]
              tunnel: w3632 -> [w3722 _ w3767 w3797]
              frame 1, Default {
                # "timeseries"
                n2185 = case shown="True" "Profile" {
                  tunnel: [w3746 w3749] -> w3727
                  tunnel: [w3746 w3748] -> w3726
                  tunnel: [w3746 w3747] -> w3725
                  tunnel: [w3746 w3751] -> w3724
                  frame False {
                    w3746 = 0.0 ("f")
                  }
                  frame True {
                    n2186 = local read "Current Position"() -> (w3750:dbl[])
                    n2187 = local read "Y change (mm)"() -> (w3751:dbl)
                    n2188 = call "subVI_explode3array.vi"("Array"=w3750) -> ("x"=w3749:dbl, "y"=w3748:dbl, "z"=w3747:dbl)  [unwired: 12 in]
                  }
                }
                n2189 = local read "Save ave N"() -> (w3745:dbl)
                n2190 = Multiply(x=w3745, y=w3738) -> (x*y=w3744:dbl)
                n2191 = To Double Precision Float(number=w3722) -> (double precision float=w3736:dbl)
                n2192 = Build Array(w3733, w3738, w3744, w3743, w3742, 0.0 ("f")) -> (w3741:dbl[])
                n2193 = Build Array(w3736, w3727, w3726, w3725, w3724) -> (w3734:dbl[])
                n2194 = Select(t=u32 4000000000, s=w3732, f="N sets to save") -> (s? t:f=w3730:u32)
                n2195 = Build Array (concatenate)(w3741, w3740, w3734) -> (w3739:dbl[])
              }
              frame 2 {
                w3755 = 0.0 ("f")
                w3752 = FALSE ("Save APD Data\nwith Trap Data")
                # "calibration"
                n2196 = Boolean To (0,1)(Boolean=w3752) -> (0, 1=w3757:i16)
                n2197 = To Double Precision Float(number=w3757) -> (double precision float=w3756:dbl)
                n2198 = Build Array(w3756, w3755, w3755, w3755, w3755) -> (w3754:dbl[])
                n2199 = Build Array(w3753, w3758, w3758, w3765, w3764, 1.0 ("t")) -> (w3762:dbl[])
                n2200 = Build Array (concatenate)(w3762, w3761, w3754) -> (w3760:dbl[])
                "Calibrating Trap..." <- TRUE ("Calibrating...")
              }
              frame 4 {
                w3772 = 0.0 ("f")
                # "write file header for a trap \nraster scan"
                # "scan dir (x/y = 0/1)"
                # "cycles/step"
                # "n scans (f/b)"
                # "steps"
                # "freq. range"
                # "AOD raster scan"
                n2201 = local read "Number of F/B Scans (AOD)"() -> (w3779:u16)
                n2202 = local read "Cycles/step (AOD)"() -> (w3781:u64)
                n2203 = local read "Scan Range (MHz)"() -> (w3784:dbl)
                n2204 = local read "Scan steps (AOD)"() -> (w3783:u64)
                n2205 = local read "Scan BD"() -> (w3791:bool)
                n2206 = local read "Save ave N"() -> (w3796:dbl)
                n2207 = Boolean To (0,1)(Boolean=w3791) -> (0, 1=w3790:i16)
                n2208 = To Double Precision Float(number=w3779) -> (double precision float=w3778:dbl)
                n2209 = To Double Precision Float(number=w3783) -> (double precision float=w3782:dbl)
                n2210 = To Double Precision Float(number=w3781) -> (double precision float=w3780:dbl)
                n2211 = To Double Precision Float(number=w3790) -> (double precision float=w3789:dbl)
                n2212 = Multiply(x=w3796, y=w3774) -> (x*y=w3795:dbl)
                n2213 = To Double Precision Float(number=w3767) -> (double precision float=w3773:dbl)
                n2214 = Build Array(w3773, w3772, w3772, w3772, w3772) -> (w3770:dbl[])
                n2215 = local read "N sets should be saved"() -> (w3776:dbl)
                n2216 = Build Array(w3789, w3784, w3782, w3780, w3778) -> (w3786:dbl[])
                n2217 = Build Array(w3769, w3774, w3795, w3794, w3793, 2.0 ("t")) -> (w3788:dbl[])
                n2218 = Round Toward +Infinity(x=w3776) -> (ceil(x): smallest int >= x=w3777:dbl)
                n2219 = Build Array (concatenate)(w3788, w3787, w3770, w3786) -> (w3785:dbl[])
                n2220 = To Unsigned Long Integer(number=w3777) -> (unsigned 32bit integer=w3775:u32)
              }
              frame 8 {
                w3805 = 0.0 ("f")
                # "MCL raster scan"
                n2221 = local read "Number of scans (MCL)"() -> (w3800:u64)
                n2222 = local read "Scan lines (y)"() -> (w3799:u64)
                n2223 = local read "2D or 1D Scan"() -> (w3802:bool)
                n2224 = local read "Scan Range (V)\n(of steps)"() -> (w3821:dbl)
                n2225 = local read "Fast Scan Dir"() -> (w3828:bool)
                n2226 = local read "Cycles/step (MCL)"() -> (w3818:u64)
                n2227 = local read "Scan steps (MCL)"() -> (w3820:u64)
                n2228 = Select(t=w3799, s=w3802, f=w3800) -> (s? t:f=w3801:u64)
                n2229 = Boolean To (0,1)(Boolean=w3802) -> (0, 1=w3804:i16)
                n2230 = local read "Save ave N"() -> (w3833:dbl)
                n2231 = local read "Initial X"() -> (w3807:dbl)
                n2232 = local read "Initial Y"() -> (w3806:dbl)
                n2233 = To Double Precision Float(number=w3804) -> (double precision float=w3803:dbl)
                n2234 = Boolean To (0,1)(Boolean=w3828) -> (0, 1=w3827:i16)
                n2235 = To Double Precision Float(number=w3801) -> (double precision float=w3816:dbl)
                n2236 = To Double Precision Float(number=w3820) -> (double precision float=w3819:dbl)
                n2237 = To Double Precision Float(number=w3818) -> (double precision float=w3817:dbl)
                n2238 = To Double Precision Float(number=w3827) -> (double precision float=w3826:dbl)
                n2239 = Multiply(x=w3833, y=w3812) -> (x*y=w3832:dbl)
                n2240 = To Double Precision Float(number=w3797) -> (double precision float=w3811:dbl)
                n2241 = local read "N sets should be saved (MCL)"() -> (w3814:dbl)
                n2242 = Build Array(w3811, w3803, w3805, w3805, w3805) -> (w3809:dbl[])
                n2243 = Build Array(w3826, w3821, w3819, w3817, w3816, w3807, w3806) -> (w3823:dbl[])
                n2244 = Build Array(w3808, w3812, w3832, w3831, w3830, 3.0 ("t")) -> (w3825:dbl[])
                n2245 = Round Toward +Infinity(x=w3814) -> (ceil(x): smallest int >= x=w3815:dbl)
                n2246 = Build Array (concatenate)(w3825, w3824, w3809, w3823) -> (w3822:dbl[])
                n2247 = To Unsigned Long Integer(number=w3815) -> (unsigned 32bit integer=w3813:u32)
              }
            }
            n2248 = local read "Index"() -> (w3672:dbl)
            n2249 = call "Create new save file.vi"("Insert"="", "Ext"=".dat", "Index In"=w3672) -> ("Path Out"=w3631:path, "Index Out"=w3644:dbl)
            n2250 = local write "Save file name"(w3631) -> ()
            n2251 = local write "Index"(w3644) -> ()
            n2252 = local write "Save index"(w3644) -> ()
            n2253 = Array Size(array=w3655) -> (size(s)=w3656:i32)
            n2254 = Open/Create/Replace File(file path (use dialog)=w3631, operation (0:open)=T24."create", access (0:read/write)=enum16{"read/write", "read-only", "write-only"}."write-only") -> (refnum out=w3669:refnum<file>)  [unwired: 1 in, 4 out]
            n2255 = local write "Saving..."(TRUE ("Saving...")) -> ()
            n2256 = To Double Precision Float(number=w3656) -> (double precision float=w3654:dbl)
            n2257 = String Length(string="Comment (data description)") -> (length=w3652:i32)
            n2258 = To Double Precision Float(number=w3652) -> (double precision float=w3651:dbl)
            n2259 = Deny Access(7:w3669) -> (3:w3668:refnum<file>)  [unwired: 1 in, 2 out]
            n2260 = Build Array (concatenate)(w3654, w3655, w3651) -> (w3653:dbl[])
            n2261 = case "If fluorescence data to be saved" shown="True" w3642 {
              tunnel: w3631 -> [_ w3721]
              tunnel: [refnum<k0> refnum w3701] -> w3643
              frame False {
              }
              frame True {
                w3700 = 0.0
                n2262 = local read "APD Integration Time (s)"() -> (w3706:dbl)
                n2263 = local read "N APD Samp/step"() -> (w3699:dbl)
                n2264 = Path To String(path=w3721) -> (string=w3720:string)
                n2265 = String Length(string=w3720) -> (length=w3719:i32)
                n2266 = Subtract(x=w3719, y=4) -> (x-y=w3717:i32)
                n2267 = String Subset(string=w3720, length (rest)=w3717) -> (substring=w3716:string)  [unwired: 1 out]
                n2268 = Build Array(w3706, w3699, w3700, w3700, w3700, w3700, w3700, w3700) -> (w3703:dbl[])
                n2269 = Concatenate Strings(w3716, "_fl.dat" ("string")) -> (w3714:string)
                n2270 = Array Size(array=w3703) -> (size(s)=w3705:i32)
                n2271 = String To Path(string=w3714) -> (path=w3710:path)
                n2272 = Open/Create/Replace File(file path (use dialog)=w3710, operation (0:open)=T24."create", access (0:read/write)=enum16{"read/write", "read-only", "write-only"}."write-only") -> (refnum out=w3711:refnum<file>)  [unwired: 1 in, 4 out]
                n2273 = Deny Access(7:w3711) -> (3:w3707:refnum<file>)  [unwired: 1 in, 2 out]
                n2274 = To Double Precision Float(number=w3705) -> (double precision float=w3704:dbl)
                n2275 = Build Array (concatenate)(w3704, w3703) -> (w3702:dbl[])
                n2276 = Write to Binary File(file (use dialog)=w3707, data=w3702, 5:FALSE ("prepend array or string size? (T)"), 9:T30."big-endian, network order" ("byte order (0:big-endian, network order)")) -> (refnum out=w3701:refnum<file>)  [unwired: 1 in, 3 out]
              }
            }
            n2277 = case shown="True" w3629 {
              tunnel: w3631 -> [_ w3683]
              tunnel: [refnum<k0> refnum w3682] -> w3630
              frame False {
              }
              frame True {
                w3678 = 0.0 ("element")
                n2278 = Path To String(path=w3683) -> (string=w3697:string)
                n2279 = Build Array(w3678, w3678, w3678, w3678, w3678, w3678, w3678, w3678) -> (w3679:dbl[])
                n2280 = String Length(string=w3697) -> (length=w3696:i32)
                n2281 = Subtract(x=w3696, y=4) -> (x-y=w3694:i32)
                n2282 = Array Size(array=w3679) -> (size(s)=w3681:i32)
                n2283 = String Subset(string=w3697, length (rest)=w3694) -> (substring=w3693:string)  [unwired: 1 out]
                n2284 = To Double Precision Float(number=w3681) -> (double precision float=w3680:dbl)
                n2285 = Concatenate Strings(w3693, "_pos.dat" ("string")) -> (w3691:string)
                n2286 = Build Array (concatenate)(w3680, w3679) -> (w3677:dbl[])
                n2287 = String To Path(string=w3691) -> (path=w3687:path)
                n2288 = Open/Create/Replace File(file path (use dialog)=w3687, operation (0:open)=T24."create", access (0:read/write)=enum16{"read/write", "read-only", "write-only"}."write-only") -> (refnum out=w3688:refnum<file>)  [unwired: 1 in, 4 out]
                n2289 = Deny Access(7:w3688) -> (3:w3684:refnum<file>)  [unwired: 1 in, 2 out]
                n2290 = Write to Binary File(file (use dialog)=w3684, data=w3677, 5:FALSE ("prepend array or string size? (T)"), 9:T30."big-endian, network order" ("byte order (0:big-endian, network order)")) -> (refnum out=w3682:refnum<file>)  [unwired: 1 in, 3 out]
              }
            }
            n2291 = Write to Binary File(file (use dialog)=w3668, data=w3653, 5:w3649, 9:w3647) -> (refnum out=w3650:refnum<file>)  [unwired: 1 in, 3 out]
            n2292 = Write to Binary File(file (use dialog)=w3650, data="Comment (data description)", 5:w3649, 9:w3647) -> (refnum out=w3646:refnum<file>)  [unwired: 1 in, 3 out]
          }
        }
        n2293 = feedback-in #19(w3589) -> ()
        n2294 = feedback-in #20(w3616) -> ()
        n2295 = feedback-in #21(w3588) -> ()
        n2296 = feedback-in #22(w3599) -> ()
        n2297 = feedback-in #23(w3602) -> ()
        n2298 = feedback-in #24(w3615) -> ()
        n2299 = feedback-in #25(w3605) -> ()
      }
      frame #1 {
        n2300 = local read "Saving..."() -> (w3846:bool)
        n2301 = case shown="True" w3846 {
          tunnel: w3850 -> [_ w3860]
          tunnel: w3849 -> [_ w3874]
          tunnel: w3848 -> [_ w3870]
          tunnel: w3847 -> [_ w3869]
          tunnel: w3845 -> [_ w3868]
          tunnel: w3844 -> [_ w3863]
          tunnel: w3843 -> [_ w3862]
          tunnel: w3842 -> [_ w3861]
          tunnel: w3841 -> [_ w3859]
          tunnel: w3840 -> [_ w3857]
          tunnel: w3839 -> [_ w3856]
          tunnel: w3838 -> [_ w3855]
          tunnel: w3837 -> [_ w3854]
          tunnel: w3836 -> [_ w3853]
          tunnel: w3835 -> [_ w3852]
          tunnel: w3834 -> [_ w3851]
          frame False {
          }
          frame True {
            n2302 = Multiply(x=w3860, y=w3859) -> (x*y=→"Time (s)":dbl)
            n2303 = Less Or Equal?(x=w3860, y=w3868) -> (x <= y?=w3872:bool)
            n2304 = Or(x="Stop Saving", y="Abort save 2") -> (x .or. y?=w3864:bool)
            n2305 = Not(x=w3864) -> (.not. x?=w3873:bool)
            n2306 = And(x=w3872, y=w3873) -> (x .and. y?=w3871:bool)
            n2307 = case shown="True" w3871 {
              tunnel: w3874 -> [w3881 w3949]
              tunnel: [0.0 w3952] -> w3867
              tunnel: w3860 -> [_ w3950]
              tunnel: w3868 -> [_ w3951]
              tunnel: w3870 -> [_ w3946]
              tunnel: w3869 -> [_ _]
              tunnel: w3863 -> [w3879 w3939]
              tunnel: w3862 -> [w3878 w3940]
              tunnel: w3861 -> [_ w3938]
              tunnel: w3857 -> [_ w3937]
              tunnel: w3856 -> [_ w3891]
              tunnel: w3855 -> [_ w3930]
              tunnel: w3854 -> [_ w3908]
              tunnel: w3853 -> [w3876 w3889]
              tunnel: w3852 -> [w3877 w3888]
              tunnel: w3851 -> [_ w3885]
              frame False {
                w3875 = FALSE
                n2308 = Close File(refnum=w3881) -> ()  [unwired: 1 in, 2 out]
                n2309 = case shown="True" w3878 {
                  tunnel: w3879 -> [_ w3883]
                  frame False {
                  }
                  frame True {
                    n2310 = Close File(refnum=w3883) -> ()  [unwired: 1 in, 2 out]
                  }
                }
                n2311 = case shown="True" w3876 {
                  tunnel: w3877 -> [_ w3882]
                  frame False {
                  }
                  frame True {
                    n2312 = Close File(refnum=w3882) -> ()  [unwired: 1 in, 2 out]
                  }
                }
                n2313 = local write "Calibrating Trap..."(w3875) -> ()
                n2314 = call <vilib>:"Beep.vi"() -> ()  [unwired: 3 in, 9 out]
                n2315 = local write "Stop Saving"(w3875) -> ()
                n2316 = property on="Raster Scanning..." class="Bool (strict)"("Val(Sgnl)"=w3875) -> ()  [unwired: 2 in, 2 out]
                "Saving..." <- w3875
              }
              frame True {
                n2317 = local read "Calibrating Trap..."() -> (w3941:bool)
                n2318 = case "Write fl. data" shown="True" w3940 {
                  tunnel: w3939 -> [_ w3975]
                  tunnel: w3938 -> [_ w3974]
                  frame False {
                  }
                  frame True {
                    n2319 = Write to Binary File(file (use dialog)=w3975, data=w3974, 5:FALSE ("prepend array or string size? (T)"), 9:T30."big-endian, network order" ("byte order (0:big-endian, network order)")) -> ()  [unwired: 1 in, 4 out]
                  }
                }
                n2320 = Greater?(x="Save ave N", y=1.0) -> (0:w3944:bool)
                n2321 = Not(x=w3941) -> (.not. x?=w3943:bool)
                n2322 = And(x=w3943, y=w3944) -> (x .and. y?=w3886:bool)
                n2323 = case shown="True" w3886 {
                  tunnel: w3885 -> [w3955 w3966]
                  tunnel: [w3955 w3958] -> w3884
                  tunnel: "Save ave N" -> [_ w3959]
                  frame False {
                  }
                  frame True {
                    w3956 = 2 ("dimension size")
                    n2324 = Array Size(array=w3966) -> (size(s)=w3960:i32)
                    n2325 = Divide(x=w3960, y=w3956) -> (x/y=w3964:dbl)
                    n2326 = Reshape Array(w3966, w3964, w3956) -> (w3965:u64[][])
